vi "LVFPGA Tx Finite Optimized.vi"(0 "device name":string="RIO0", 1 "Enabled Channels":string(combo)="0", 5 "IQ rate":dbl=10000000.0 caption="IQ Rate" format="%#.3pS/s", 7 "number of samples":i64=16384 caption="Number of Samples", 9 "run duration":dbl=5.0 format="%#_13g", 11 "error in":errorcluster) -> (6 "coerced IQ rate":dbl format="%#_6p", 8 "underflow":bool, 10 "overflow":bool, 15 "error out":errorcluster)   [LabVIEW 2015]
doc: "This template is for the Simple NI-USRP Streaming design, a design that shows the basics of streaming data to an NI USRP-294x/295x device. Refer to the block diagram for more information about how to use this template."
uses:
  SubVIs/niusrprios Start Trigger.ctl
  SubVIs/niusrprios Configure Signal (Level).vi
  SubVIs/niusrprios Write Tx Data (I16 multi).vi
  SubVIs/niusrprios Generate Waveform (Interleaved).vi
panel:
  out "iterations":i32
  out "error out before clear":errorcluster
  in  "which bitfile":string(combo)="Time"
  in  "Reference Frequency Source":string(combo)="Internal"
  out "generating":bool caption="Generating"
  in  "stop":bool
  # "Tx Streaming"
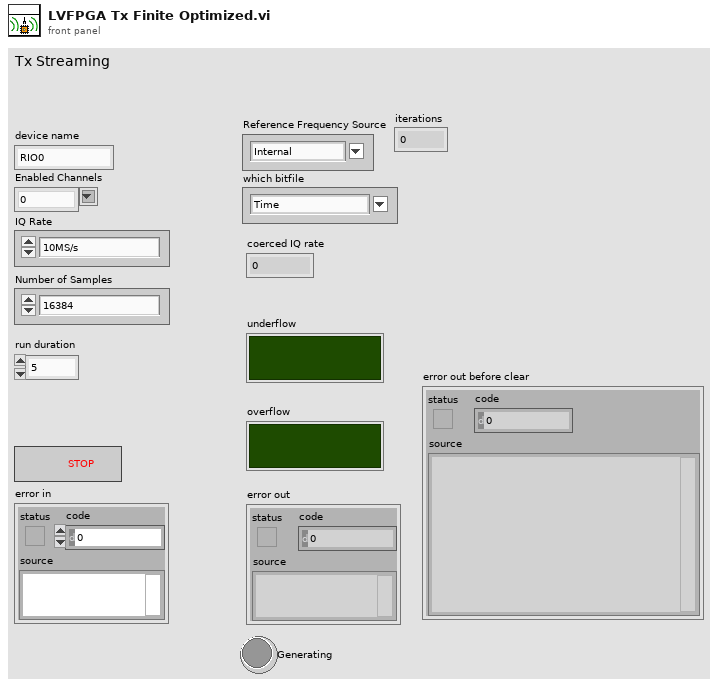
[diagram p1: front panel]
types:
  T1 = typedef "niusrprios Start Trigger.ctl" = enum8{"Software", "Digital Edge", "Rx Start Trigger", "Tx Start Trigger", "Immediate", "Future Time Event"}
  T2 = cluster{"antenna":string, "frequency":dbl, "lo frequency":dbl, "level":dbl}
  T3 = cluster{"channel enable":bool, "channel configuration":cluster{"antenna":string, "frequency":dbl, "lo frequency":dbl, "level":dbl}}
  T4 = cluster{"antenna":string, "frequency":dbl, "lo frequency":dbl, "level":dbl}[]
  T5 = typedef "niUsrpRio Config v1 Host.lvlib/niUsrpRio Session.ctl" = cluster{"FPGA Interface":refnum<k20>, "RIO Interface Number":u32, "Data Clock Rate":u32, "FPGA Data Clock Rate":u32, "Global Settings Register Bus":T6, "Radio 0 Settings Register Bus":T6, "Radio 1 Settings Register Bus":T6, "Radio Settings Bus Semaphore":T7, "DB Queues":T8[], "Characterization Data Valid?":bool, "EEPROM Header":T9, "Device Data Header":T10, "EEPROM Characterization Header":T11, "Characterization Data":T12[], "FPGA Current Version":u32, "FPGA Oldest Compatible Version":u32, "Fixed Logic Current Version":u32, "Fixed Logic Oldest Compatible Version":u32, "FPGA Radio Settings Bus Current Version":u32, "FPGA Radio Settings Bus Oldest Compatible Version":u32, "FPGA Board Config Current Version":u32, "FPGA Board Config Oldest Compatible Version":u32, "Daughterboard Clock Rate":u32}
  T6 = typedef "niInstr Register Bus v0 Host.lvlib/Register Bus Session.ctl" = refnum<queue>
  T7 = typedef "Semaphore RefNum" = refnum<k1>
  T8 = typedef "niUsrpRio Config v1 Host.lvlib/DB Queue Reference.ctl" = refnum<queue>
  T9 = typedef "niUsrpRio Config v1 Host.lvlib/EEPROM Header.ctl" = cluster{"Checksum":u32, "Product Code":u16, "Hardware Current Version":u16, "Hardware Oldest Compatible Version":u16, "EEPROM Map Current Version":u16, "EEPROM Map Oldest Compatible Version":u16, "User Password":string, "Pointer to Factory Header":u32, "Pointer to User Header":u32, "Recommended Interval":u16, "Number of Reserved Bytes":i32, "Number of Daughterboards":u8, "Daughterboard IDs":u16[], "Daughterboard Serial Numbers":string[]}
  T10 = typedef "niUsrpRio Config v1 Host.lvlib/EEPROM Device Data Header.ctl" = cluster{"Checksum":u32, "Number of Channels":u8, "Number of Gain Settings":u16[], "Pointer to Characterization Data":u32[], "Number of Reserved Bytes":i32, "Number of Frequencies":u16[]}
  T11 = typedef "niUsrpRio Config v1 Host.lvlib/EEPROM Characterization Header.ctl" = cluster{"Checksum":u32, "Date":timestamp, "Temperature":sgl, "Misc. Info":string, "Pointer to Device Data Header":u32, "Number of Reserved Bytes":i32}
  T12 = typedef "niUsrpRio Config v1 Host.lvlib/Characterization Data.ctl" = cluster{"Gains[dB]":dbl[], "Frequencies [Hz]":dbl[], "IQ Imbalance Table":T13[], "Measured Gains[dB]":dbl[][]}
  T13 = typedef "niUsrpRio Config v1 Host.lvlib/IQ Imbalance.ctl" = cluster{"Gain Imbalance [linear]":dbl, "Phase Imbalance [radians]":dbl, "Offset":cdb}
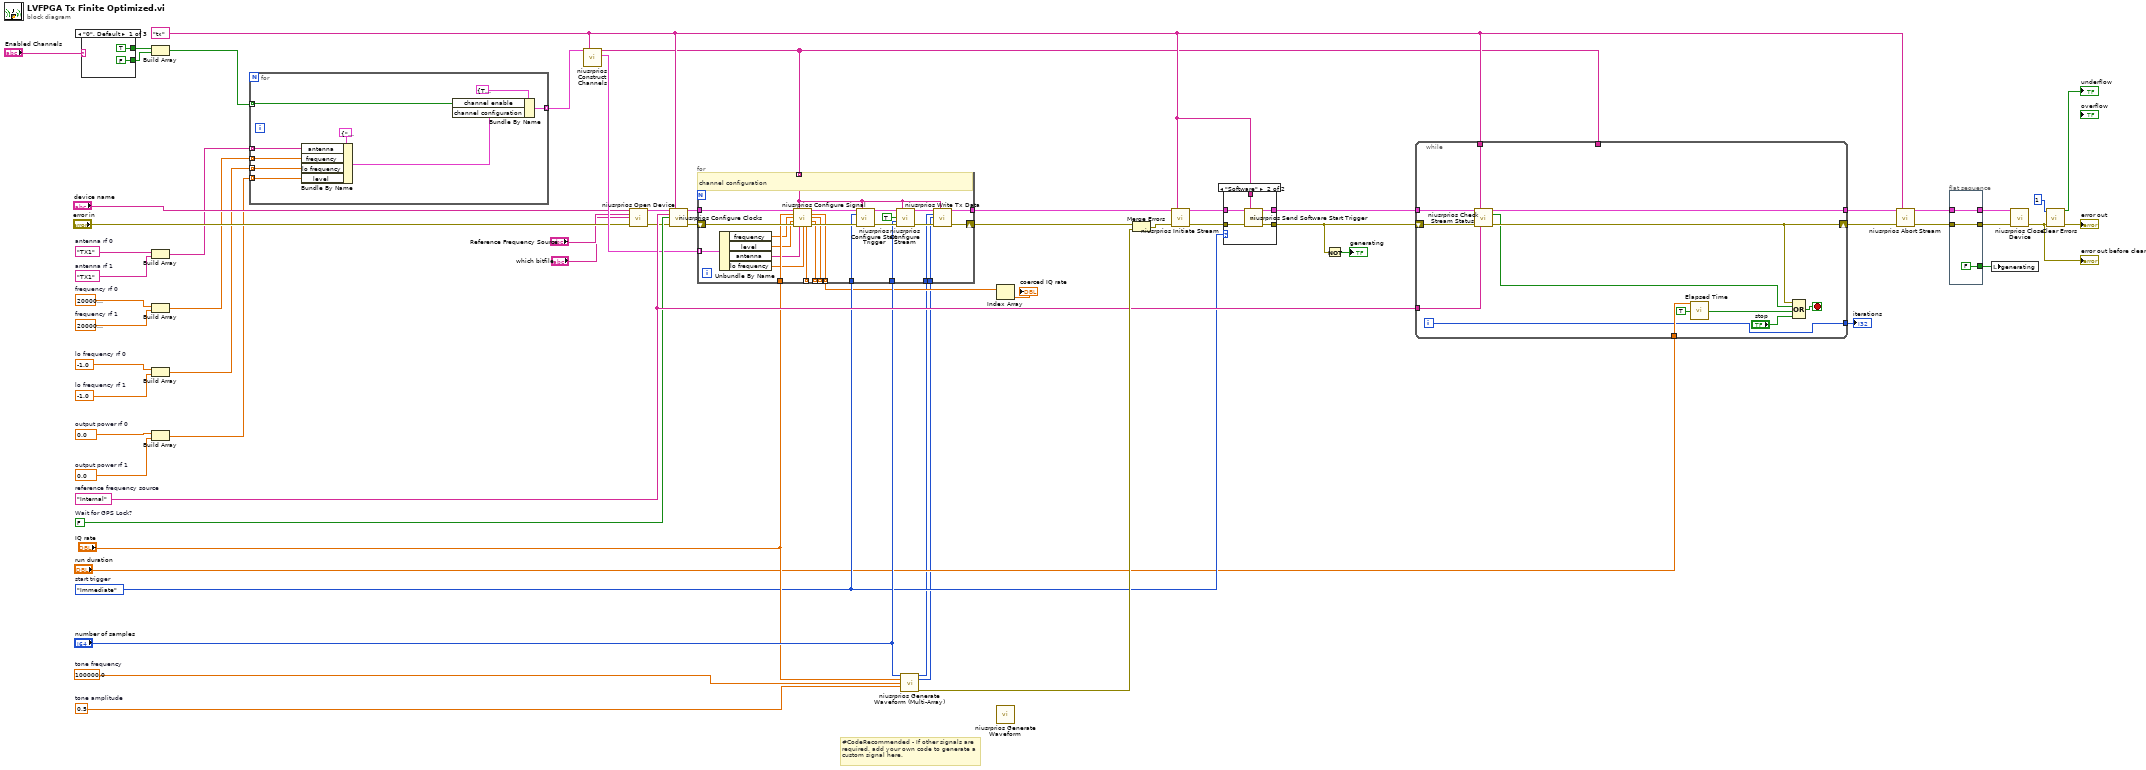
[diagram p0: block diagram]
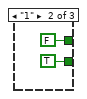
[diagram p2: hidden frame]
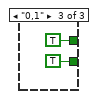
[diagram p3: hidden frame]
diagram:
  w47 = 100000.0  # tone frequency
  w38 = niusrprios_Start_Trigger."Immediate"  # start trigger
  w60 = "Internal"  # reference frequency source
  w51 = 0.0  # output power rf 1
  w50 = 0.0  # output power rf 0
  w52 = -1.0  # lo frequency rf 1
  w53 = -1.0  # lo frequency rf 0
  w54 = 2000000000.0  # frequency rf 1
  w55 = 2000000000.0  # frequency rf 0
  w57 = "TX1"  # antenna rf 1
  w56 = "TX1"  # antenna rf 0
  w39 = FALSE  # Wait for GPS Lock?
  w46 = 0.5  # tone amplitude
  w34 = "tx" ("scope")
  # "#CodeRecommended - If other signals are required, add your own code to generate a custom signal here."
  n1 = case shown="\"0\", Default" "Enabled Channels" {
    tunnel: [TRUE FALSE TRUE] -> w20
    tunnel: [FALSE TRUE TRUE] -> w19
    frame "0", Default {
    }
    frame "1" {
    }
    frame "0,1" {
    }
  }
  n2 = Build Array(w20, w19) -> (w12:bool[])
  n3 = Build Array(w56, w57) -> (w11:string[])
  n4 = Build Array(w55, w54) -> (w10:dbl[])
  n5 = Build Array(w53, w52) -> (w9:dbl[])
  n6 = Build Array(w50, w51) -> (w8:dbl[])
  n7 = for {
    tunnel: w12 -> [w75] mode=indexing
    tunnel: w11 -> [w73] mode=indexing
    tunnel: w10 -> [w72] mode=indexing
    tunnel: w9 -> [w71] mode=indexing
    tunnel: w8 -> [w70] mode=indexing
    tunnel: [w68] -> w7 mode=indexing
    n8 = Bundle By Name(cluster=T2 {"antenna"="", "frequency"=0.0, "lo frequency"=0.0, "level"=0.0} ("channel configuration"), "antenna"=w73, "frequency"=w72, "lo frequency"=w71, "level"=w70) -> (w69:T2)
    n9 = Bundle By Name(cluster=T3 {"channel enable"=TRUE, "channel configuration"={"antenna"="RX1", "frequency"=2000000000.0, "lo frequency"=-1.0, "level"=0.0}} ("channel configuration"), "channel enable"=w75, "channel configuration"=w69) -> (w68:T3)
  }
  n10 = call "niusrprios Construct Channels.vi"("channel configurations"=w7, "scope"=w34) -> ("enabled channels"=w33:string[], "enabled channel configurations"=w32:T4)  [unwired: 12 in]
  n11 = call "niusrprios Open Device.vi"("USRP RIO device"="device name", "Reference Frequency Source"="Reference Frequency Source", "which bitfile"="which bitfile", "error in"="error in") -> ("niUsrpRio Session (out)"=w31:T5, "error out"=w30:errorcluster)  [unwired: 10 in]
  n12 = call "niusrprios Configure Clocks.vi"("niUsrpRio Session"=w31, "scope"=w34, "Reference Frequency Source"=w60, "GPSDO Power Enable"=w39, "error in"=w30) -> ("niUsrpRio Session (out)"=w28:T5, "error out"=w29:errorcluster)  [unwired: 9 in]
  n13 = call "niusrprios Generate Waveform (Multi-Array).vi"("number of samples"="number of samples", "sample rate"="IQ rate", "tone frequency"=w47, "amplitude"=w46) -> ("I"=w4:i16[], "Q"=w3:i16[], "error out"=w61:errorcluster)  [unwired: 8 in, 1 out]
  n14 = for {
    tunnel: [w86] -> _ mode=indexing
    tunnel: [w91] -> w26
    tunnel: w38 -> [w100]
    tunnel: "number of samples" -> [w95]
    shift-right: [w93] -> w25
    shift-left: w29 -> [w96]
    tunnel: w33 -> [w90] mode=indexing
    tunnel: "IQ rate" -> [w94]
    tunnel: w3 -> [w89]
    tunnel: w4 -> [w88]
    tunnel: w28 -> [w87]
    tunnel: [w85] -> _ mode=indexing
    tunnel: [w84] -> _ mode=indexing
    tunnel: [w83] -> w23 mode=indexing
    tunnel: w32 -> [w82] mode=indexing
    # "channel configuration"
    n15 = Unbundle By Name(w82) -> ("frequency"=w81:dbl, "level"=w80:dbl, "antenna"=w79:string, "lo frequency"=w78:dbl)
    n16 = call-poly "niusrprios Configure Signal.vi"("niUsrpRio Session"=w87, "scope"=w90, "sample rate [S/s]"=w94, "frequency [Hz]"=w81, "level [dBm]"=w80, "error in"=w96, "Active Antenna"=w79, "LO frequency [Hz]"=w78) -> ("niUsrpRio Session (out)"=w98:T5, "coerced sample rate [S/s]"=w83:dbl, "coerced frequency [Hz]"=w84:dbl, "coerced level [dBm]"=w85:dbl, "coerced LO frequency [Hz]"=w86:dbl, "error out"=w102:errorcluster)  [unwired: 1 in, 1 out]
    n17 = call "niusrprios Configure Start Trigger.vi"("niUsrpRio Session"=w98, "scope"=w90, "start trigger"=w100, "error in"=w102) -> ("niUsrpRio Session (out)"=w97:T5, "error out"=w99:errorcluster)  [unwired: 10 in]
    n18 = call "niusrprios Configure Stream.vi"("niUsrpRio Session"=w97, "scope"=w90, "number of samples is finite"=TRUE, "number of samples"=w95, "error in"=w99) -> ("niUsrpRio Session (out)"=w92:T5, "error out"=w101:errorcluster)  [unwired: 9 in]
    n19 = call-poly "niusrprios Write Tx Data.vi"("niUsrpRio Session"=w92, "scope"=w90, "I"=w88, "Q"=w89, "error in"=w101) -> ("niUsrpRio Session (out)"=w91:T5, "error out"=w93:errorcluster)  [unwired: 9 in]
  }
  n20 = Index Array(array=w23) -> (element=→"coerced IQ rate":dbl)  [unwired: 1 in]
  n21 = call-poly "niusrprios Generate Waveform.vi"() -> ()  [unwired: 13 in, 3 out]
  n22 = Merge Errors(w25, w61) -> (w24:errorcluster)
  n23 = call "niusrprios Initiate Stream.vi"("niUsrpRio Session"=w26, "scope"=w34, "error in"=w24) -> ("niUsrpRio Session (out)"=w35:T5, "error out"=w36:errorcluster)  [unwired: 11 in]
  n24 = case shown="\"Software\"" w38 {
    tunnel: w36 -> [w104 w109]
    tunnel: [w104 w108] -> w37
    tunnel: w35 -> [w103 w107]
    tunnel: w34 -> [_ w106]
    tunnel: [w103 w105] -> w27
    frame Default {
    }
    frame "Software" {
      n25 = call "niusrprios Send Software Start Trigger.vi"("niUsrpRio Session"=w107, "scope"=w106, "error in"=w109) -> ("niUsrpRio Session (out)"=w105:T5, "error out"=w108:errorcluster)  [unwired: 11 in]
    }
  }
  n26 = Not(x=w37) -> (.not. x?=→"generating":bool)
  n27 = while {
    tunnel: [w113] -> w59
    tunnel: w33 -> [_]
    tunnel: w27 -> [w120]
    tunnel: w34 -> [w118]
    tunnel: w60 -> [w117]
    tunnel: "run duration" -> [w114]
    shift-right: [w112] -> w58
    shift-left: w37 -> [w119]
    tunnel: [w110] -> w1
    i -> [w110]
    stop <- w122 stop-if-true
    # "Acquire and Fetch a waveform"
    n28 = call "niusrprios Check Stream Status.vi"("niUsrpRio Session"=w120, "scope"=w118, "error in"=w119, "reference frequency source"=w117) -> ("niUsrpRio Session (out)"=w113:T5, "done"=w111:bool, "error out"=w112:errorcluster)  [unwired: 9 in]
    n29 = call "Elapsed Time"("Time Target (s)"=w114, "Auto Reset"=TRUE) -> ("Time has Elapsed"=w115:bool)  [unwired: 10 in, 7 out]
    n30 = Compound Arithmetic op=OR(w112, w111, w115, "stop") -> (w122:bool)
  }
  "iterations" <- w1
  n31 = call "niusrprios Abort Stream.vi"("niUsrpRio Session"=w59, "scope"=w34, "error in"=w58) -> ("niUsrpRio Session (out)"=w44:T5, "error out"=w45:errorcluster)  [unwired: 11 in]
  n32 = flat-sequence {
    tunnel: [w125] -> w43
    tunnel: w44 -> [w125]
    tunnel: [w124] -> w42
    tunnel: w45 -> [w124]
    tunnel: [FALSE ("Generating")] -> w41
    frame #0 {
    }
  }
  n33 = local write "generating"(w41) -> ()
  n34 = call "niusrprios Close Device.vi"("niUsrpRio Session"=w43, "error in"=w42) -> ("error out"=w2:errorcluster)  [unwired: 13 in]
  "error out before clear" <- w2
  n35 = call <vilib>:"Clear Errors.vi"("error in (no error)"=w2, "specific error code to clear (0: all)"=1) -> ("error out"=→"error out":errorcluster, "specific error cleared?"=→"underflow":bool)  [unwired: 4 in]
